vi "PM100D_Read_ph.vi"(2 "stop":bool, 3 "Beam Name":string, 4 "Wavelength (0.0)":sgl=533.0) -> (0 "error out":errorcluster, 1 "Average Power (mW)":dbl)   [LabVIEW 2020]
uses:
  <vilib>/Instr/_visa.llb/VISA Find Search Mode.ctl
panel:
  out "Sensor Flags":i16
  out "Sensor Type":i16
  out "Sensor Subtype":i16
  out "Sensor Calibration Message":string
  out "Sensor Name":string
  out "Sensor Serial Number":string
  out "Waveform Chart":dbl(graph)
  out "String":string
  out "Current Power (mW)":dbl caption="Power" format="%_4f"
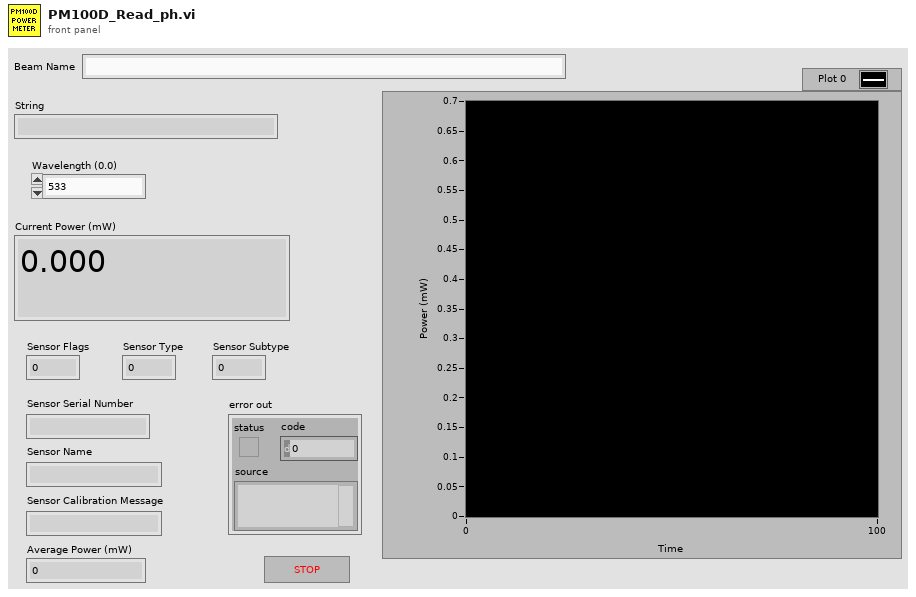
[diagram p1: front panel]
types:
  T1 = typedef "VISA Find Search Mode.ctl" = u32
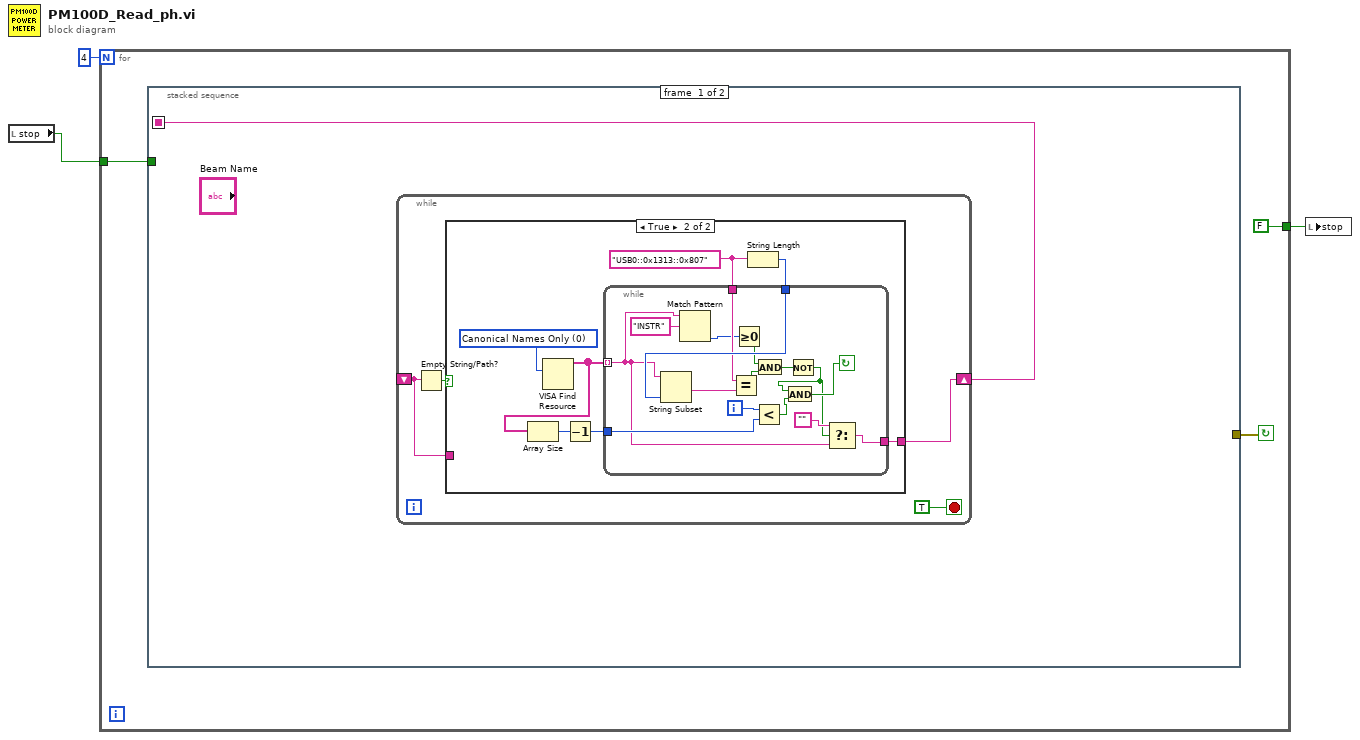
[diagram p0: block diagram]
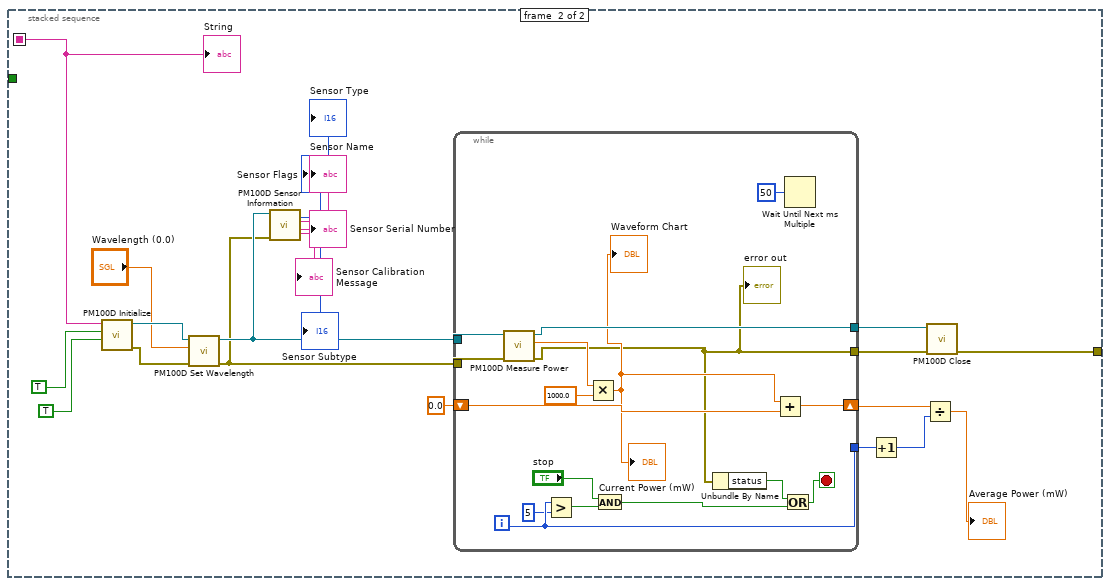
[diagram p3: hidden frame]
diagram:
  n1 = local read "stop"() -> (w3:bool)
  n2 = for {
    N: 4 -> [_]
    tunnel: w3 -> [w5]
    tunnel: [FALSE ("stop")] -> w1
    stop <- w6 continue-if-true
    n3 = stacked-sequence {
      seq-local: [w7 _] -> [_ w52]
      tunnel: [_ w36] -> w6
      tunnel: w5 -> [_ _]
      frame #0 {
        n4 = while {
          shift-right: [w11] -> w7
          shift-left: _ -> [w9]
          stop <- TRUE stop-if-true
          n5 = Empty String/Path?(string/path=w9) -> (empty?=w10:bool)
          n6 = case shown="True" w10 {
            tunnel: [w12 w13] -> w11
            tunnel: w9 -> [w12 _]
            frame False {
            }
            frame True {
              w19 = T1 0 items=["Canonical Names Only"=0, "Aliases Only"=1, "Include Matching Aliases"=2, "Include All Aliases"=4] ("Search Mode")
              w17 = "USB0::0x1313::0x807" ("element")
              n7 = VISA Find Resource(10:w19) -> (3:w16:string[])  [unwired: 1 in, 3 out]
              n8 = Array Size(array=w16) -> (size(s)=w15:i32)
              n9 = Decrement(x=w15) -> (x-1=w14:i32)
              n10 = String Length(string=w17) -> (length=w18:i32)
              n11 = while {
                tunnel: w18 -> [w35]
                tunnel: w16 -> [w25] mode=indexing
                tunnel: w17 -> [w34]
                tunnel: w14 -> [w31]
                tunnel: [w28] -> w13
                i -> [w32]
                stop <- w29 continue-if-true
                n12 = String Subset(string=w25, length (rest)=w35) -> (substring=w33:string)  [unwired: 1 in]
                n13 = Match Pattern(string=w25, regular expression="INSTR") -> (offset past match=w24:i32)  [unwired: 1 in, 3 out]
                n14 = Equal?(x=w34, y=w33) -> (x = y?=w22:bool)
                n15 = Greater Or Equal To 0?(x=w24) -> (x >= 0?=w23:bool)
                n16 = Less?(x=w32, y=w31) -> (x < y?=w30:bool)
                n17 = And(x=w23, y=w22) -> (x .and. y?=w21:bool)
                n18 = Not(x=w21) -> (.not. x?=w20:bool)
                n19 = And(x=w20, y=w30) -> (x .and. y?=w29:bool)
                n20 = Select(t="", s=w20, f=w25) -> (s? t:f=w28:string)
              }
            }
          }
        }
      }
      frame #1 {
        n21 = call "PM100D Initialize.vi"("Reset Device (Reset Device)"=TRUE, "ID Query (Do Query)"=TRUE, "resource name"=w52) -> ("error out"=w54:errorcluster, "instrument handle out"=w55:refnum<visa-resource-name>)  [unwired: 7 in]
        n22 = call "PM100D Set Wavelength.vi"("error in (no error)"=w54, "Wavelength (0.0)"="Wavelength (0.0)", "instrument handle"=w55) -> ("error out"=w49:errorcluster, "instrument handle out"=w50:refnum<visa-resource-name>)  [unwired: 7 in]
        n23 = call "PM100D Sensor Information.vi"("error in (no error)"=w49, "instrument handle"=w50) -> ("Sensor Serial Number"=→"Sensor Serial Number":string, "Sensor Name"=→"Sensor Name":string, "Sensor Calibration Message"=→"Sensor Calibration Message":string, "Sensor Type"=→"Sensor Type":i16, "Sensor Subtype"=→"Sensor Subtype":i16, "Sensor Flags"=→"Sensor Flags":i16)  [unwired: 2 in, 2 out]
        n24 = while {
          tunnel: w50 -> [w74]
          tunnel: w49 -> [w73]
          tunnel: [w58] -> w37
          tunnel: [w72] -> w51
          shift-right: [w71] -> w40
          shift-left: 0.0 -> [w70]
          tunnel: [w66] -> w41
          i -> [w66]
          stop <- w60 stop-if-true
          n25 = call "PM100D Measure Power.vi"("error in (no error)"=w73, "instrument handle"=w74) -> ("error out"=w58:errorcluster, "Power"=w68:dbl, "instrument handle out"=w72:refnum<visa-resource-name>)  [unwired: 7 in]
          "error out" <- w58
          n26 = Greater?(x=w66, y=5) -> (0:w64:bool)
          n27 = Multiply(x=w68, y=1000.0) -> (x*y=w67:dbl)
          "Current Power (mW)" <- w67
          "Waveform Chart" <- w67
          n28 = And(x="stop", y=w64) -> (x .and. y?=w61:bool)
          n29 = Unbundle By Name(w58) -> ("status"=w62:bool)
          n30 = Add(x=w67, y=w70) -> (x+y=w71:dbl)
          n31 = Or(x=w62, y=w61) -> (x .or. y?=w60:bool)
          n32 = Wait Until Next ms Multiple(millisecond multiple=u32 50) -> ()  [unwired: 1 out]
        }
        n33 = Increment(x=w41) -> (x+1=w39:i32)
        n34 = Divide(x=w40, y=w39) -> (x/y=→"Average Power (mW)":dbl)
        n35 = call "PM100D Close.vi"("error in (no error)"=w37, "instrument handle"=w51) -> ("error out"=w36:errorcluster)  [unwired: 9 in]
        "String" <- w52
      }
    }
  }
  n36 = local write "stop"(w1) -> ()
